vi "AVI-Set to AVI1 mode.vi"() -> (3 "AVI mode":T1)   [LabVIEW 2020]
uses:
  Typedefs/AVI implementation enum.ctl
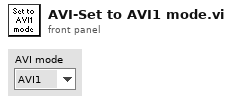
[diagram p1: front panel]
types:
  T1 = typedef "AVI implementation enum.ctl" = enum16{"AVI1", "AVI2"}
  T2 = enum16{"Write Red AVI", "Write Green AVI", "Write AVI mode"}
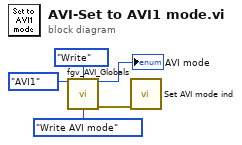
[diagram p0: block diagram]
diagram:
  n1 = call "fgv_AVI_Globals.vi"("AVI mode"=AVI_implementation_enum."AVI1", "Function"=enum16{"Intialize", "Write", "Read", "Clear"}."Write", "\"Write\" sub function"=T2."Write AVI mode" ("\"Write\" sub function")) -> ("AVI mode"=→"AVI mode":T1, "error out"=w2:errorcluster)  [unwired: 9 in, 2 out]
  n2 = call "Set AVI mode ind.vi"("error in (no error)"=w2) -> ()  [unwired: 10 in, 1 out]
